vi "Measurement Data Convert (Normal).vi"(8 "error in (no error)":errorcluster, 9 "Item Number Offset (1)":i32=1 min=1 max=255, 10 "Measurement Data (Empty)":string, 11 "VISA resource name":refnum<visa-resource-name>) -> (0 "error out":errorcluster, 1 "Measurement":dbl[](array[numeric]), 2 "Function":string[](array[string]), 3 "VISA resource name out":refnum<visa-resource-name>)   [LabVIEW 2018, in "Yokogawa WT300 Series.lvlib"]
doc: "Transforms measurement datas into normal numeric values."
uses:
  Yokogawa WT300 Series.lvlib
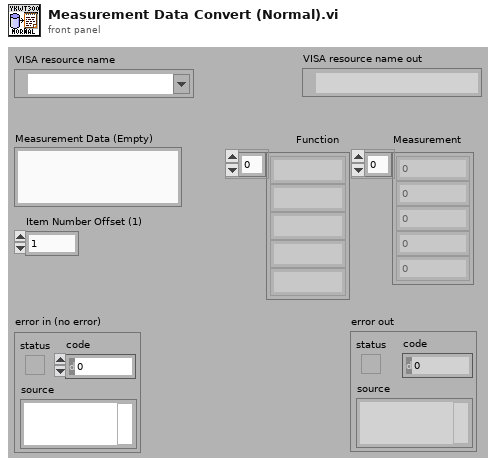
[diagram p1: front panel]
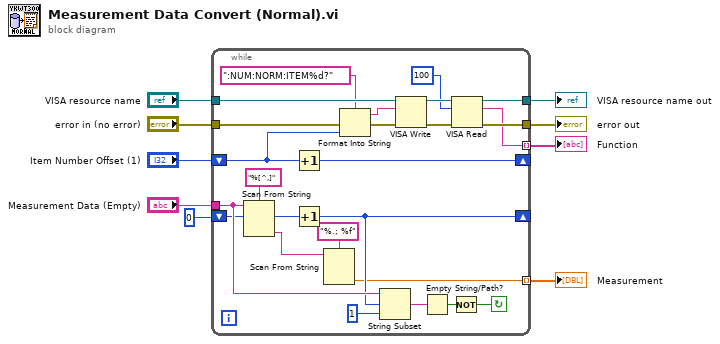
[diagram p0: block diagram]
diagram:
  n1 = while {
    tunnel: [w24] -> w3 mode=indexing
    tunnel: "Measurement Data (Empty)" -> [w29]
    shift-right: [w26] -> _
    shift-left: 0 -> [w28]
    tunnel: "VISA resource name" -> [w21]
    tunnel: "error in (no error)" -> [w18]
    shift-right: [w22] -> _
    shift-left: "Item Number Offset (1)" -> [w11]
    tunnel: [w19] -> w6
    tunnel: [w15] -> w5
    tunnel: [w14] -> w4 mode=indexing
    stop <- w31 continue-if-true
    n2 = Scan From String(format string="%[^,]", input string=w29, initial scan location=w28) -> (offset past scan=w27:u32, output 1=w25:string)  [unwired: 2 in, 2 out]
    n3 = Increment(x=w11) -> (x+1=w22:i32)
    n4 = Increment(x=w27) -> (x+1=w26:u32)
    n5 = Scan From String(format string="%.; %f" ("Œ`Ž®•¶Žš—ñ"), input string=w25) -> (output 1=w24:dbl)  [unwired: 3 in, 3 out]
    n6 = Format Into String(format string=":NUM:NORM:ITEM%d?" ("Œ`Ž®•¶Žš—ñ"), error in=w18, w11) -> (resulting string=w10:string, error out=w17:errorcluster)  [unwired: 1 in]
    n7 = String Subset(string=w29, offset (0)=w26, length (rest)=1) -> (substring=w33:string)
    n8 = VISA Write ("VISA書き込み")(VISA resource name=w21, write buffer=w10, error in (no error)=w17) -> (VISA resource name out=w20:refnum<visa-resource-name>, error out=w16:errorcluster)  [unwired: 1 out]
    n9 = Empty String/Path?(string/path=w33) -> (empty?=w32:bool)
    n10 = Not(x=w32) -> (.not. x?=w31:bool)
    n11 = VISA Read ("VISA読み取り")(VISA resource name=w20, byte count=u32 100, error in (no error)=w16) -> (VISA resource name out=w19:refnum<visa-resource-name>, read buffer=w14:string, error out=w15:errorcluster)  [unwired: 1 out]
  }
  "error out" <- w5
  "VISA resource name out" <- w6
  "Measurement" <- w3
  "Function" <- w4
